vi "WPI_DigitalModuleSetRelayForward.vi"(8 "error in (no error)":errorcluster, 9 "Value":bool, 10 "RelayChannel":T1, 11 "DigitalModuleDevRef":T2) -> (0 "error out":errorcluster, 3 "DigitalModuleDevRef":T2)   [LabVIEW 2017]
doc: "This software is licensed. Open the labview\\readme\\WPI Robotics Library Open Source License.txt file for more information."
uses:
  <vilib>/Rock Robotics/WPI/DigitalModule/WPI_DigitalModuleDeviceRef.ctl
  <vilib>/Rock Robotics/SystemInterfaces/DIO/FPGA_DIORelayChannel.ctl
  <vilib>/Rock Robotics/SystemInterfaces/System/FPGA_SystemGet.vi
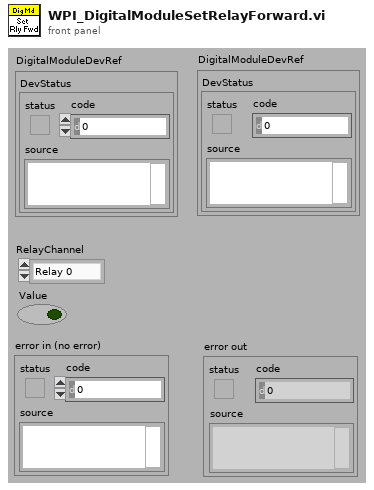
[diagram p1: front panel]
types:
  T1 = typedef "FPGA_DIORelayChannel.ctl" = enum8{"Relay 0", "Relay 1", "Relay 2", "Relay 3", "Invalid"}
  T2 = typedef "WPI_DigitalModuleDeviceRef.ctl" = cluster{"DevStatus":errorcluster}
  T3 = typedef "FPGA_DIODevRef.ctl" = cluster{"DevStatus":errorcluster}
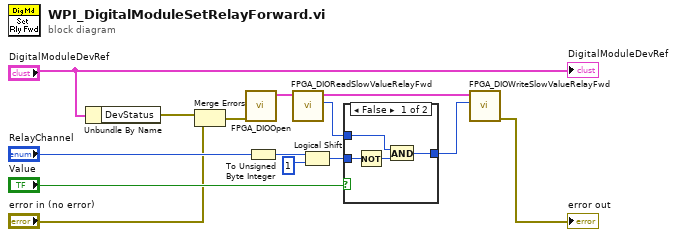
[diagram p0: block diagram]
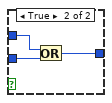
[diagram p2: hidden frame]
diagram:
  n1 = Unbundle By Name("DigitalModuleDevRef") -> ("DevStatus"=w4:errorcluster)
  n2 = Merge Errors(w4, "error in (no error)") -> (w3:errorcluster)
  n3 = call <vilib>:"FPGA_DIOOpen.vi"("error in (no error)"=w3) -> ("DIODeviceRef"=w11:T3)  [unwired: 1 in, 9 out]
  n4 = To Unsigned Byte Integer(number="RelayChannel") -> (unsigned 8bit integer=w6:u8)
  n5 = call <vilib>:"FPGA_DIOReadSlowValueRelayFwd.vi"("DIODeviceRef In"=w11) -> ("Relay Forward"=w8:u8, "DIODeviceRef Out"=w10:T3)  [unwired: 1 in, 8 out]
  n6 = Logical Shift(y=w6, x=u8 1) -> (x << y=w5:u8)
  n7 = case shown="False" "Value" {
    tunnel: w8 -> [w16 w20]
    tunnel: w5 -> [w18 w21]
    tunnel: [w15 w19] -> w9
    frame False {
      n8 = Not(x=w18) -> (.not. x?=w17:u8)
      n9 = And(x=w16, y=w17) -> (x .and. y?=w15:u8)
    }
    frame True {
      n10 = Or(x=w20, y=w21) -> (x .or. y?=w19:u8)
    }
  }
  n11 = call <vilib>:"FPGA_DIOWriteSlowValueRelayFwd.vi"("Relay Forward"=w9, "DIODeviceRef In"=w10) -> ("error out"=→"error out":errorcluster)  [unwired: 1 in, 8 out]
  "DigitalModuleDevRef" <- "DigitalModuleDevRef"
